vi "FPGA Config.vi"() -> ()   [LabVIEW 2013]
uses:
  <vilib>/rvi/Emulation/niFpgaSctlEmulationGetInTimedLoop.vi
  <vilib>/rvi/Emulation/niFpgaEmulationReportErrorSimple.vi
  <vilib>/rvi/Emulation/niFpgaGetClockAttributes.vi
  <vilib>/rvi/eio/common/nirviEmuTemplateMethod_errors.vi
  <vilib>/rvi/Emulation/niFpgaCriticalErrorInLSC.vi
  <vilib>/eio/EIONode/EIONode.xnode
panel:
  in  "Pulse Width(uSec)":i32 caption="Pulse Width (mSec)"
  out "ModA/AI3":fxp<+/-,26,5>
  out "ModA/AI2":fxp<+/-,26,5>
  out "ModA/AI1":fxp<+/-,26,5>
  in  "Count(mSec)":u32=50
  in  "stop":bool
  out "ModA/AI0":fxp<+/-,26,5>
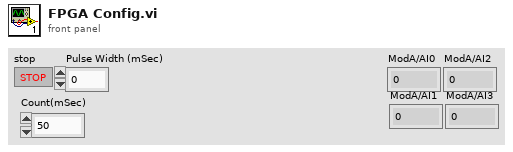
[diagram p1: front panel]
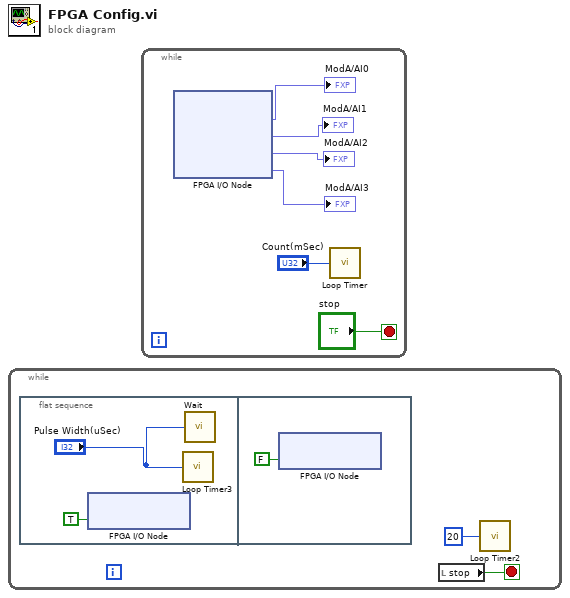
[diagram p0: block diagram]
diagram:
  n1 = while {
    stop <- w1 stop-if-true
    n2 = flat-sequence {
      frame #0 {
        n3 = xnode "FPGA I/O Node"("Port5/DIO9"=TRUE) -> ()  [unwired: 1 in, 1 out]
        n4 = call "Loop Timer3"("Count(uSec)"="Pulse Width(uSec)") -> ()  [unwired: 1 out]
        n5 = call "Wait"("Count(uSec)"="Pulse Width(uSec)") -> ()  [unwired: 1 out]
      }
      frame #1 {
        n6 = xnode "FPGA I/O Node"("Port5/DIO9"=FALSE) -> ()  [unwired: 1 in, 1 out]
      }
    }
    n7 = local read "stop"() -> (w1:bool)
    n8 = call "Loop Timer2"("Count(mSec)"=u32 20) -> ()  [unwired: 1 out]
  }
  n9 = while {
    stop <- "stop" stop-if-true
    n10 = xnode "FPGA I/O Node"() -> ("ModA/AI0"=→"ModA/AI0":fxp<+/-,26,5>, "ModA/AI1"=→"ModA/AI1":fxp<+/-,26,5>, "ModA/AI2"=→"ModA/AI2":fxp<+/-,26,5>, "ModA/AI3"=→"ModA/AI3":fxp<+/-,26,5>)  [unwired: 4 in, 4 out]
    n11 = call "Loop Timer"("Count(mSec)"="Count(mSec)") -> ()  [unwired: 1 out]
  }
